vi "Image to Info.vi"(8 "error in (no error)":errorcluster, 10 "Child Indexes":i32[](array[numeric]), 11 "Image in":T3) -> (0 "error out":errorcluster, 3 "JSON Image out":T1)   [LabVIEW 2026]
uses:
  <vilib>/picture/picture.llb/imagedata.ctl
  Controls/JSON Image Data.ctl
  Controls/Image Position.ctl
  <vilib>/wsapi/NI_WebServices.lvlib
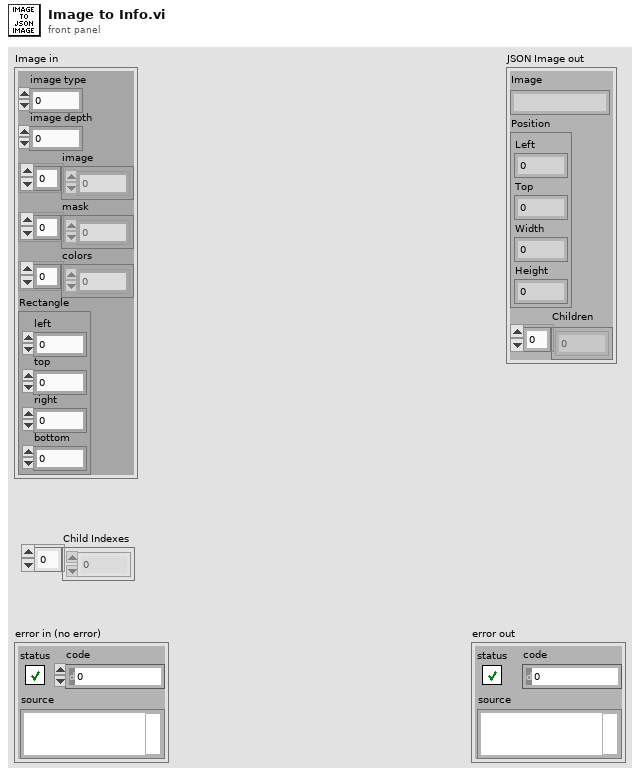
[diagram p1: front panel]
types:
  T1 = typedef "JSON Image Data.ctl" = cluster{"Image":string, "Position":T2, "Children":dbl[]}
  T2 = typedef "Image Position.ctl" = cluster{"Left":i16, "Top":i16, "Width":i16, "Height":i16}
  T3 = typedef "imagedata.ctl" = cluster{"image type":i32, "image depth":i32, "image":u8[], "mask":u8[], "colors":u32[], "Rectangle":cluster{"left":i16, "top":i16, "right":i16, "bottom":i16}}
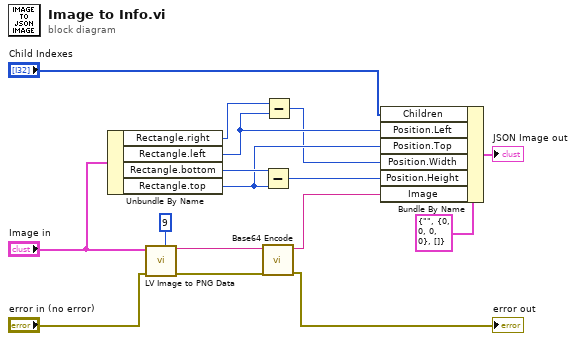
[diagram p0: block diagram]
diagram:
  n1 = Unbundle By Name("Image in") -> ("Rectangle.right"=w12:i16, "Rectangle.left"=w6:i16, "Rectangle.bottom"=w13:i16, "Rectangle.top"=w5:i16)
  n2 = call <vilib>:"LV Image to PNG Data.vi"("compression (none)"=9, "error in (no error)"="error in (no error)", "image data"="Image in") -> ("error out"=w9:errorcluster, "png data"=w11:string)  [unwired: 7 in]
  n3 = Subtract(x=w13, y=w5) -> (x-y=w4:i16)
  n4 = call "Base64 Encode.vi"("error in (no error)"=w9, "string in (not encoded)"=w11) -> ("error out"=→"error out":errorcluster, "string out (base64-encoded)"=w10:string)  [unwired: 8 in]
  n5 = Subtract(x=w12, y=w6) -> (x-y=w3:i16)
  n6 = Bundle By Name(cluster=T1 {"Image"="", "Position"={"Left"=0, "Top"=0, "Width"=0, "Height"=0}, "Children"=[]} ("JSON Image out"), "Children"="Child Indexes", "Position.Left"=w6, "Position.Top"=w5, "Position.Width"=w3, "Position.Height"=w4, "Image"=w10) -> (→"JSON Image out":T1)
